vi "氨氮MB_api.vi"(6 "Slave ID":u8=1, 7 "STEP":enum16{"open", "read", "write", "close"}(ring)=enum."read", 8 "Error in":errorcluster caption="Error in (no error)", 9 "values":u16[](array[numeric]), 10 "quantity":u16, 11 "starting address":u16 format="%04xH") -> (0 "error out":errorcluster, 1 "MB session out":refnum<class "MB_Master.lvclass">, 2 "MB_TCP session":refnum<class "MB_Master_TCP.lvclass">, 3 "Registers":u16[](array[numeric]))   [LabVIEW 2016, in "斯坦道氨氮.lvlib"]
uses:
  <vilib>/Plasmionique/MB Master/MB_Master/MB_Master.lvclass
  <vilib>/Plasmionique/MB Master/MB_Master_TCP/MB_Master_TCP.lvclass
  D:/Program Files (x86)/National Instruments/LabVIEW 2016/vi.lib/Plasmionique/MB Master/MB_Master/MB_Master.lvclass
  <vilib>/Plasmionique/MB Master/MB_Master_Serial/MB_Master_Serial.lvclass
  <vilib>/Plasmionique/MB Master/MB Master.lvlib
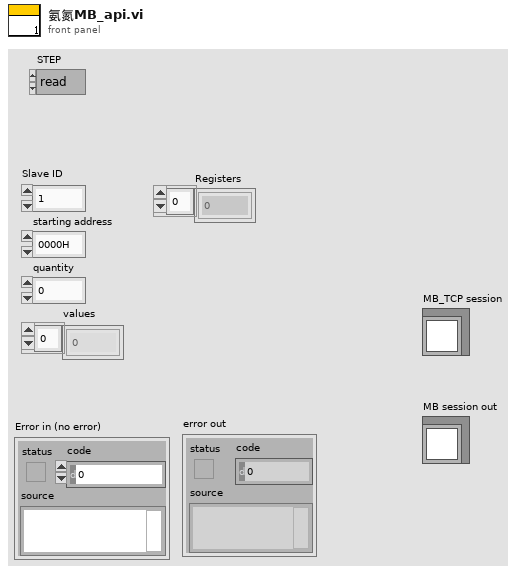
[diagram p1: front panel]
types:
  T1 = cluster{"baud rate (bps)":u32, "stop bits":u16, "parity":u16, "flow control":u16, "timeout":u32, "retries":i32}
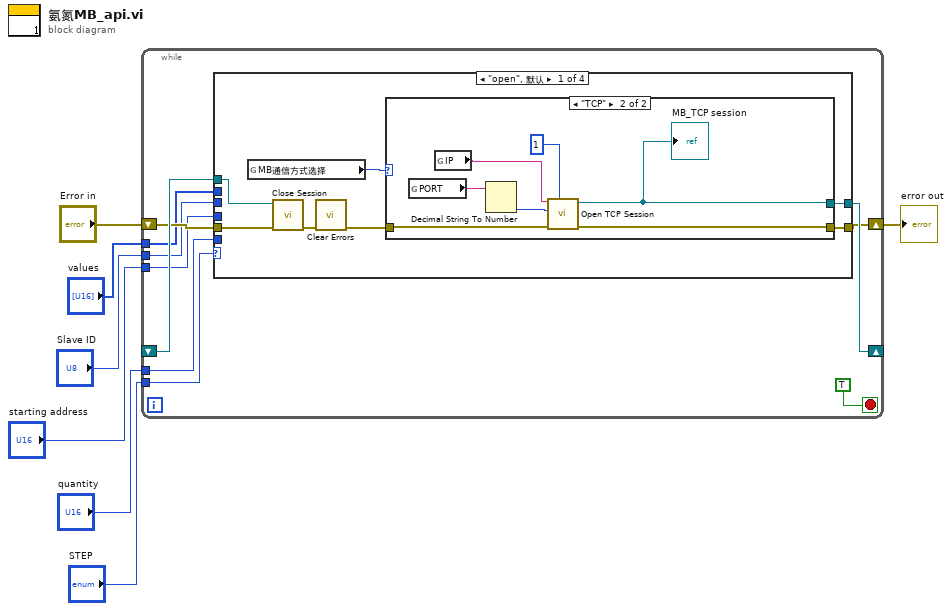
[diagram p0: block diagram]
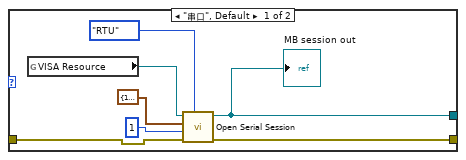
[diagram p2: hidden frame]
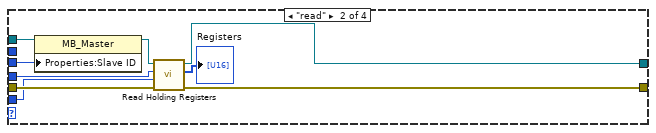
[diagram p3: hidden frame]
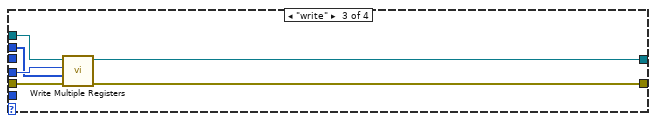
[diagram p4: hidden frame]
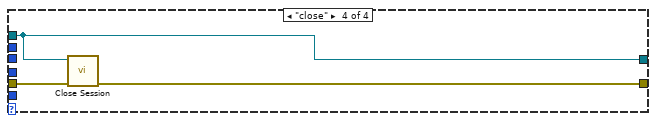
[diagram p5: hidden frame]
diagram:
  n1 = while {
    shift-right: [w9] -> _
    shift-left: _ -> [w17]
    shift-right: [w8] -> w6
    shift-left: "Error in" -> [w16]
    tunnel: "Slave ID" -> [w15]
    tunnel: "starting address" -> [w14]
    tunnel: "quantity" -> [w13]
    tunnel: "STEP" -> [w12]
    tunnel: "values" -> [w11]
    stop <- TRUE stop-if-true
    n2 = case shown="\"open\", 默认" w12 {
      tunnel: w17 -> [w24 w40 w51 w54]
      tunnel: w16 -> [w23 w47 w53 w56]
      tunnel: [w20 w46 w50 w54] -> w9
      tunnel: [w19 w45 w52 w55] -> w8
      tunnel: w15 -> [_ w43 _ _]
      tunnel: w14 -> [_ w42 w49 _]
      tunnel: w13 -> [_ w41 _ _]
      tunnel: w11 -> [_ _ w48 _]
      frame "open", Default {
        n3 = global read "氨氮断电保存全局变量.vi" "MB通信方式选择"() -> (w18:enum16{"串口", "TCP"})
        n4 = call-dynamic "Close Session.vi"("error in (no error)"=w23, "MB session in"=w24) -> ("error out"=w22:errorcluster)  [unwired: 9 in]
        n5 = call <vilib>:"Clear Errors.vi"("error in (no error)"=w22) -> ("error out"=w21:errorcluster)  [unwired: 5 in, 1 out]
        n6 = case shown="\"TCP\"" w18 {
          tunnel: [w31 w37] -> w19
          tunnel: [w30 w36] -> w20
          tunnel: w21 -> [w25 w35]
          frame "串口", Default {
            n7 = global read "氨氮断电保存全局变量.vi" "VISA Resource"() -> (w28:refnum<visa-resource-name>)
            n8 = call <vilib>:"Open Serial Session.vi"("Mode (RTU)"=enum16{"RTU", "ASCII"}."RTU", "Error in"=w25, "Slave ID"=u8 1, "Serial Config"=T1 {"baud rate (bps)"=115200, "stop bits"=10, "parity"=0, "flow control"=0, "timeout"=100, "retries"=1}, "VISA Resource"=w28) -> ("Error out"=w31:errorcluster, "MB_Serial session"=w30:refnum<class "MB_Master_Serial.lvclass">)  [unwired: 5 in]
            "MB session out" <- w30
          }
          frame "TCP" {
            n9 = global read "氨氮断电保存全局变量.vi" "PORT"() -> (w33:string)
            n10 = global read "氨氮断电保存全局变量.vi" "IP"() -> (w34:string)
            n11 = Decimal String To Number(string=w33) -> (number=w38:i32)  [unwired: 2 in, 1 out]
            n12 = call <vilib>:"Open TCP Session.vi"("Slave ID (255)"=u8 1 ("Slave ID"), "error in (no error)"=w35, "Port (502)"=w38, "IP Address"=w34) -> ("error out"=w37:errorcluster, "MB_TCP session"=w36:refnum<class "MB_Master_TCP.lvclass">)  [unwired: 6 in]
            "MB_TCP session" <- w36
          }
        }
      }
      frame "read" {
        n13 = property class="MB_Master"(reference=w40, "Properties:Slave ID"=w43) -> (reference out=w39:refnum<class "MB_Master.lvclass">)  [unwired: 1 in, 1 out]
        n14 = call <vilib>:"Read Holding Registers.vi"("error in (no error)"=w47, "quantity"=w41, "starting address"=w42, "MB session in"=w39) -> ("error out"=w45:errorcluster, "Registers"=→"Registers":u16[], "MB session out"=w46:refnum<class "MB_Master.lvclass">)  [unwired: 5 in]
      }
      frame "write" {
        n15 = call <vilib>:"Write Multiple Registers.vi"("error in (no error)"=w53, "values"=w48, "starting address"=w49, "MB session in"=w51) -> ("error out"=w52:errorcluster, "MB session out"=w50:refnum<class "MB_Master.lvclass">)  [unwired: 6 in]
      }
      frame "close" {
        n16 = call-dynamic "Close Session.vi"("error in (no error)"=w56, "MB session in"=w54) -> ("error out"=w55:errorcluster)  [unwired: 9 in]
      }
    }
  }
  "error out" <- w6
